vi "Problem 4 - Largest palindrome product.vi"() -> ()   [LabVIEW 2021, in "Project Euler.lvlib"]
uses:
  Project Euler.lvlib
  Utilities/Numeric Utilities/Numeric Utilities.lvlib
panel:
  out "No. of elements in B":i32
  out "Palindrome products only (array B)":i32[](array[numeric])
  out "No. of elements in A":i32
  out "All products of two 3-digit numbers (array A)":i32[](array[numeric])
  out "Answer":i32
  # "Development\nControls or indicators that are useful for development or testing, but which are not outputs of the VI."
  # "Input\nInputs to the VI"
  # "Output\nOutputs of the VI"
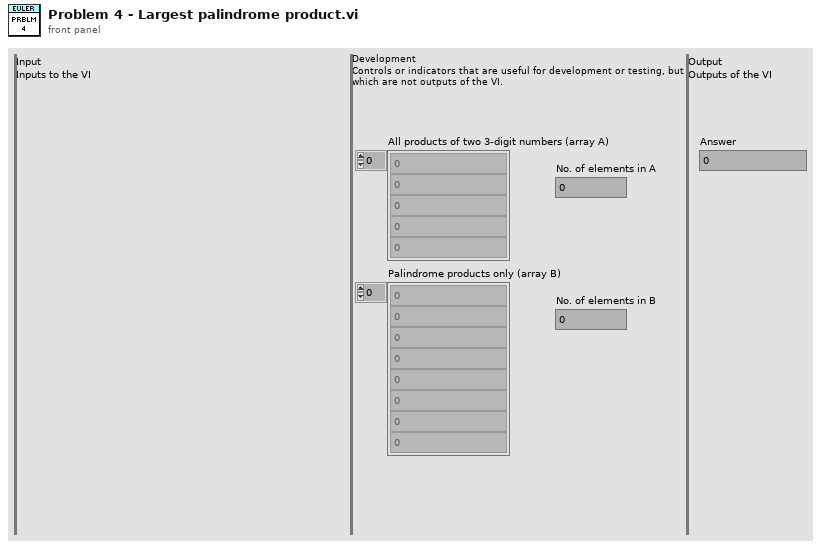
[diagram p1: front panel]
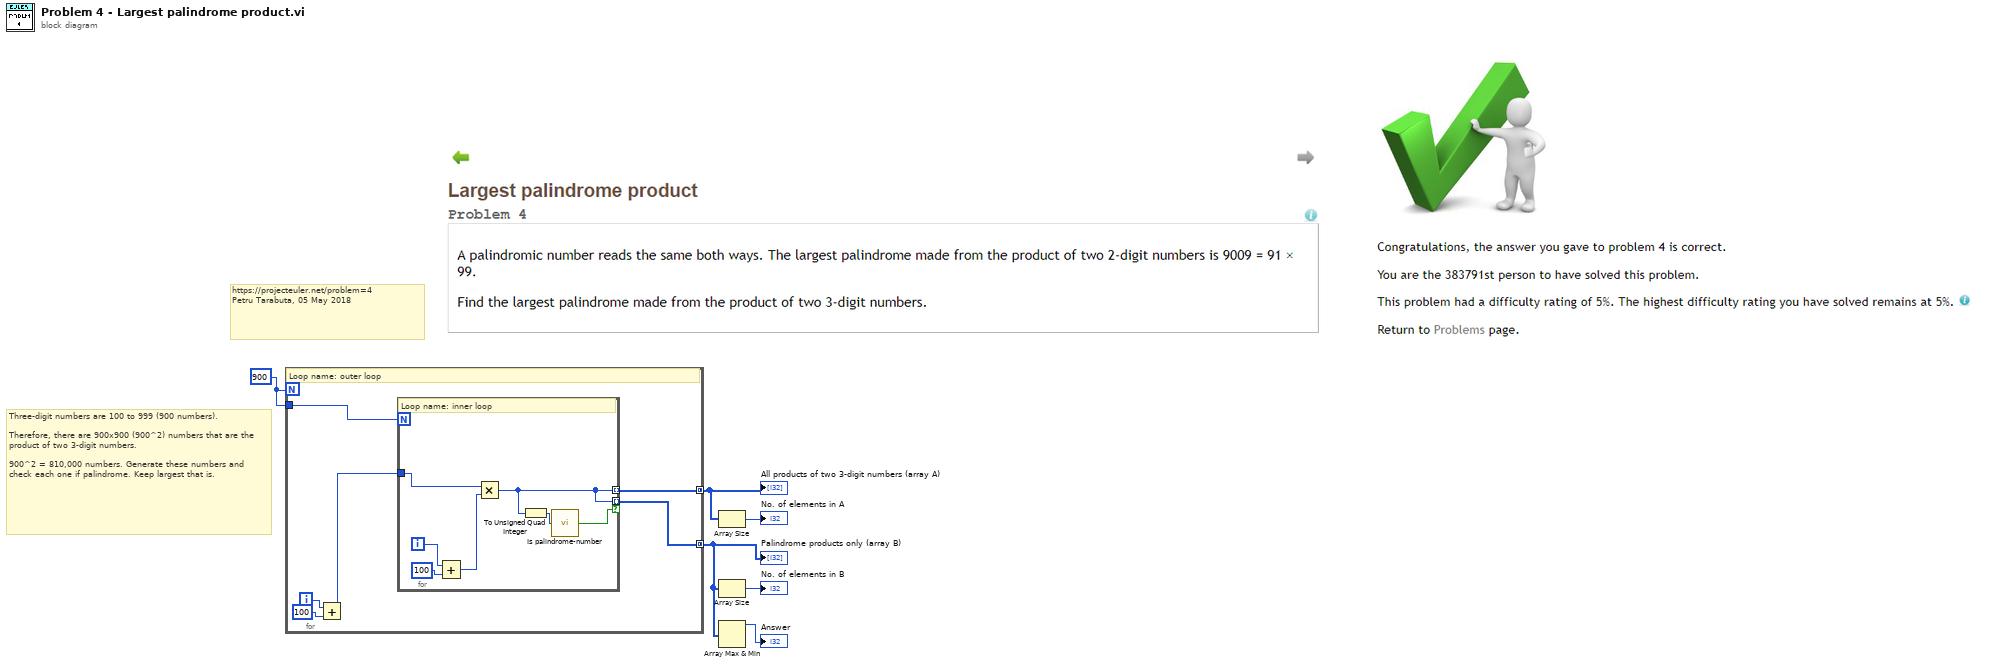
[diagram p0: block diagram]
diagram:
  w6 = 900
  # "Three-digit numbers are 100 to 999 (900 numbers).\n\nTherefore, there are 900x900 (900^2) numbers that are the product of two 3-digit numbers.\n\n900^2 = 810,000 numbers. Generate these numbers and check each one if palindrome. Keep largest that is."
  # "https://projecteuler.net/problem=4\nPetru Tarabuta, 05 May 2018"
  n1 = for {
    N: w6 -> [_]
    tunnel: w6 -> [w10]
    tunnel: [w8] -> w5 mode=concatenating
    tunnel: [w7] -> w2 mode=concatenating
    i -> [w12]
    # "Loop name: outer loop"
    n2 = Add(x=w12, y=100) -> (x+y=w9:i32)
    n3 = for {
      N: w10 -> [_]
      tunnel: w9 -> [w17]
      tunnel: [w14] -> w8 mode=indexing
      tunnel: [w14] -> w7 mode=indexing if=w13
      i -> [w18]
      # "Loop name: inner loop"
      n4 = Add(x=w18, y=100) -> (x+y=w16:i32)
      n5 = Multiply(x=w17, y=w16) -> (x*y=w14:i32)
      n6 = To Unsigned Quad Integer(1:w14) -> (0:w15:u64)
      n7 = call "Is palindrome-number.vi"("x"=w15) -> ("T = x is a palindrome"=w13:bool)
    }
  }
  "All products of two 3-digit numbers (array A)" <- w5
  "Palindrome products only (array B)" <- w2
  n8 = Array Size(array=w5) -> (size(s)=→"No. of elements in A":i32)
  n9 = Array Size(array=w2) -> (size(s)=→"No. of elements in B":i32)
  n10 = Array Max & Min(array=w2) -> (max value=→"Answer":i32)  [unwired: 3 out]
